vi "fgv_udp_config_remote.vi"(7 "cmd":enum16{"write", "read"}(ring)=enum."read", 8 "error in":errorcluster, 11 "udp cfg":T1={"local port"=61556, "remote port"=61550, "RBA IP"="192.168.1.109"}) -> (0 "error out":errorcluster, 3 "udp cfg out":T1={"local port"=61556, "remote port"=61550, "RBA IP"="192.168.1.109"})   [LabVIEW 2019]
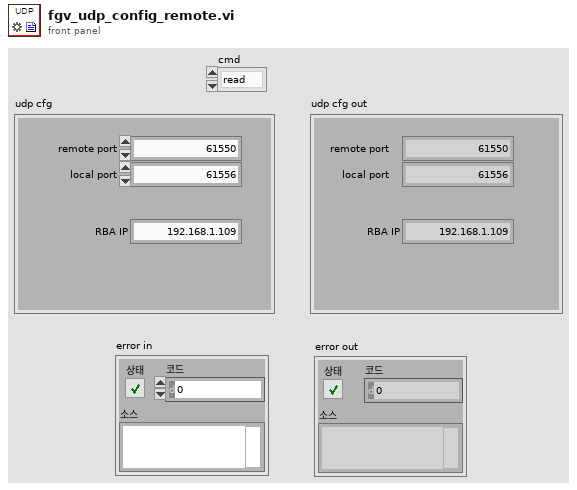
[diagram p1: front panel]
types:
  T1 = cluster{"local port":u16, "remote port":u16, "RBA IP":string}
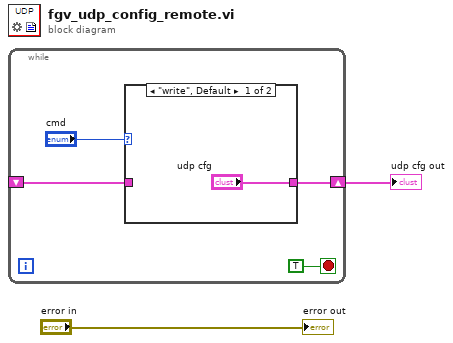
[diagram p0: block diagram]
diagram:
  n1 = while {
    shift-right: [w4] -> w2
    shift-left: _ -> [w3]
    stop <- TRUE stop-if-true
    n2 = case shown="\"write\", Default" "cmd" {
      tunnel: ["udp cfg" w8] -> w4
      tunnel: w3 -> [_ w8]
      frame "write", Default {
      }
      frame "read" {
      }
    }
  }
  "udp cfg out" <- w2
  "error out" <- "error in"
